vi "Set JSON Value.vi"(8 "error in (no error)":errorcluster, 9 "File Contents":string="{\n    \"SMUResourceName\": \"SMU1\",\n    \"SMUChannels\": \"0\",\n\t\"SMUSourceMode_Sequence\": 1021,\n\t\"SMUOutputFunction_DCCurrent\": 1007,\n    \"SMUSourceTransientResponse_Fast\": 1039,\n    \"SMUCurrent\": 1.0,\n    \"SMUCurrentLevelRange\": 1.0,\n    \"SMUMeasurementSense_Local\": 1008,\n    \"SMUMeasurementApertureTime\": 0.010,\n    \"SMUSourceAdvancedSourceDelay\": 0.000100,\n    \"SMUVoltage\": 6,\n    \"SMUSourceAdvancedSequenceLoopCount\": 571,\n    \"SMUMeasurementAdvancedDCNoiseRejection_Normal\": 1044,\n\t\"SMUSequenceName\": \"MySequence\",\n\t\"SMUStep1_Source_DCCurrent_CurrentLevel\": 1150009,\n\t\"SMUStep2_Measurement_ApertureTime\": 1150058,\n\t\"SMUStep3_Source_Advanced_SourceDelay\": 1150051,\n\t\"SMUSequenceNumberOfSteps\": 3,\n\t\"SMUTriggerFromSwitch_StartDigitalEdge\": \"/SMU/PXI_Trig1\",\n\t\"SMUTriggerFromSwitch_SequenceAdvanceDigitalEdge\": \"/SMU/PXI_Trig1\",\n\t\"SMUTriggerToDMM_SourceCompleteEvent\": 1030,\n\t\"SMUTriggerToDMM_SourceCompleteEvent_Value\": \"/SMU/PXI_Trig2\",\n\t\"SMUTriggerToSwitch_SequenceIterationCompleteEvent\": 1032,\n\t\"SMUTriggerToDMM_SequenceIterationCompleteEvent_Value\": \"/SMU/PXI_Trig0\",\n\t\n\t\"Switch1ResourceName\": \"2526_1\",\n\t\"Switch1Topology\": \"2526/2-Wire 79x1 Mux\",\n\t\"Switch1ScanList\": \"ch70:75->com\",\n\t\n\t\"Switch2ResourceName\": \"SwitchBlock1Dev1\",\n\t\"Switch2Topology\": \"Configured Topology\",\n\t\"Switch2ScanList\": \"[c2->card1r2->c26], [c3->card1r3->c27]; [c6->card1r2->c26], [c7->card1r3->c27]; [c10->card1r2->c26], [c11->card1r3->c27]; [c14->card1r2->c26], [c15->card1r3->c27]; [c18->card1r2->c26], [c19->card1r3->c27]; [c22->card1r2->c26], [c23->card1r3->c27];\",\n\t\n\t\"DMMResourceName\": \"DMM\",\n\t\"DMMFunction_DCVolts\": 0,\n\t\"DMMResolution\": 0.1,\n\t\"DMMRange\": 0.1,\n\t\"DMMTriggerSource_TTL2\": 4,\n\t\"DMMTriggerSlope_RisingEdge\": 0,\n\t\"DMMSampleTrigger_TTL2\": 4,\n\t\"DMMSampleCount\": 0,\n\t\"DMMSampleTriggerSlope_RisingEdge\": 0,\n\t\"DMMApertureTimeUnits_Seconds\": 0,\n\t\"DMMApertureTime\": 0.010,\n\t\"DMMNumberOfAverages\": 1,\n\t\"DMMAutoZero_Off\": 0,\n\t\"DMMADCCalibration_Off\": 0,\n\t\"DMMSettleTime\": 0.0001,\n\t\"DMMControlAction_Commit\": 0,\n\t\n\t\"ApplicationNumberOfWeldChannels\": 6\n}", 10 "Parameter and Value":string="SETCONF=SMUResourceName[[CONFPARAM]]=SMU", 11 "JSON Configuration File (.json)":path=path "C:/Users/chericks/Desktop/JSONtest/labview-grpc-query-server/jsontestfile2.json") -> (0 "error out":errorcluster)   [LabVIEW 2019]
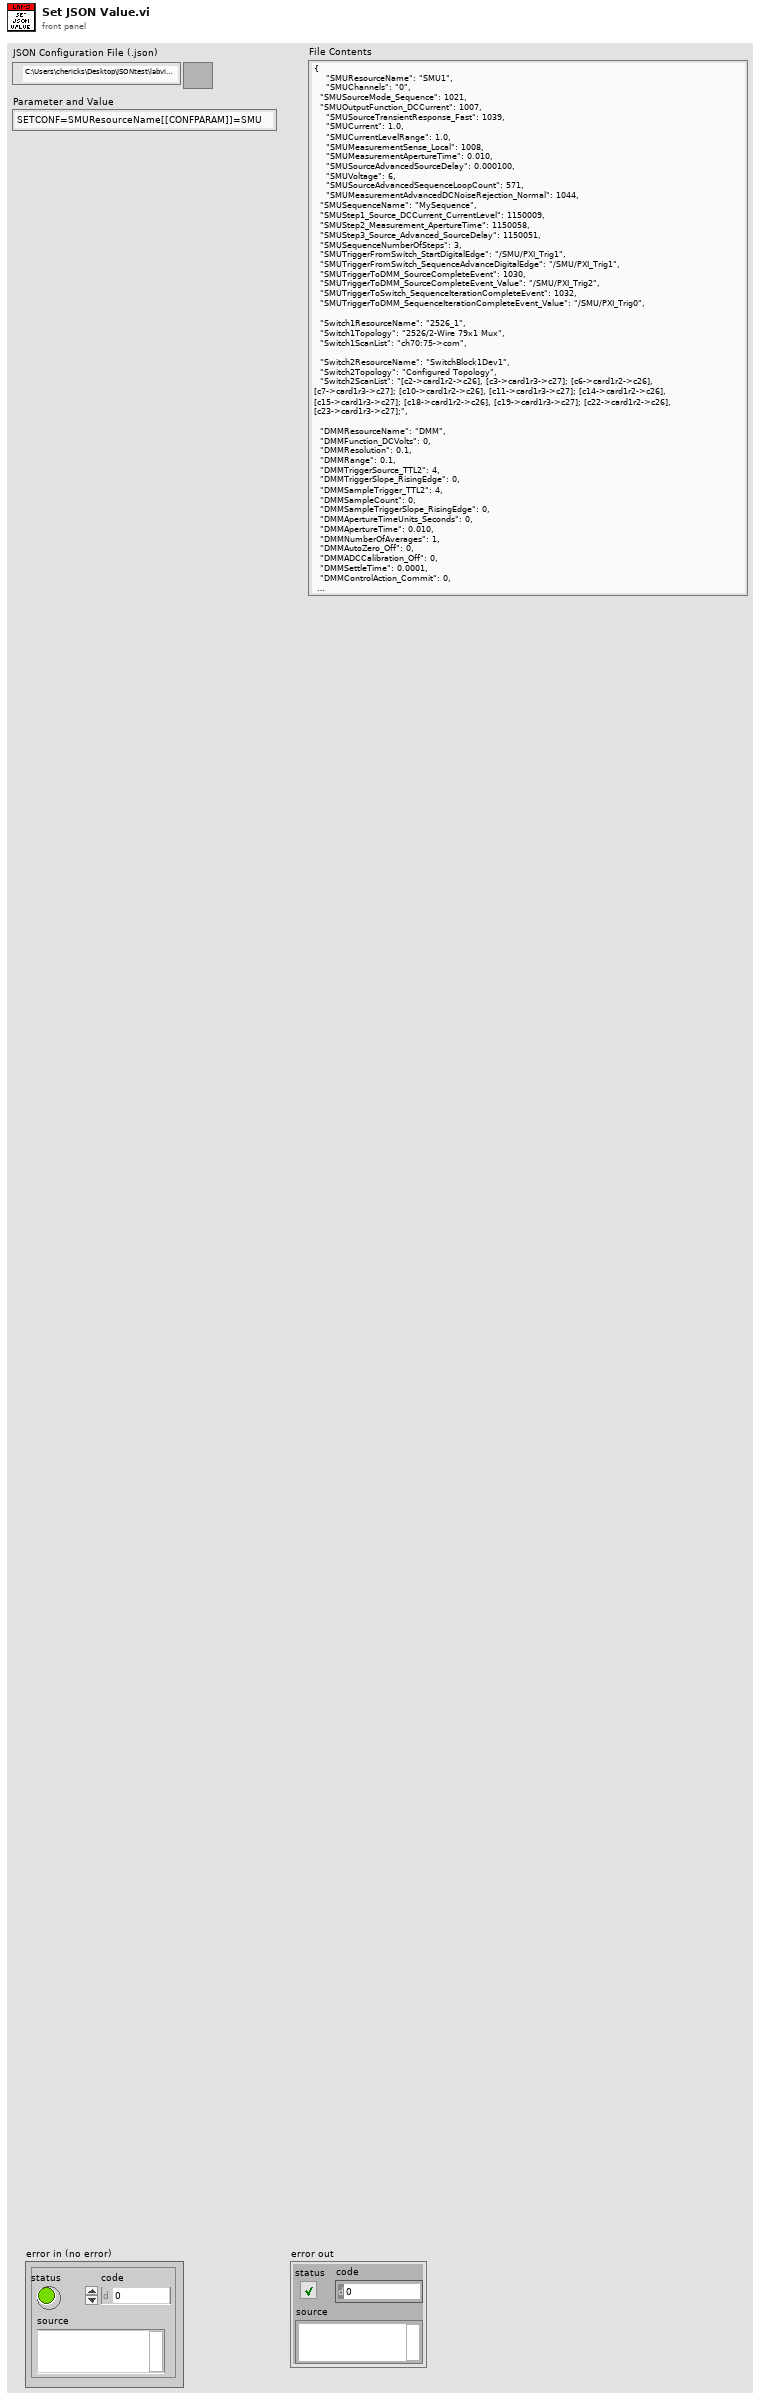
[diagram p1: front panel]
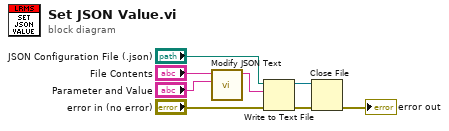
[diagram p0: block diagram]
diagram:
  n1 = call "Modify JSON Text.vi"("Parameter and Value"="Parameter and Value", "JSONtextin"="File Contents") -> ("JSONtextout"=w2:string)  [unwired: 9 in]
  n2 = Write to Text File(file (use dialog)="JSON Configuration File (.json)", text=w2, error in="error in (no error)") -> (refnum out=w5:refnum<file>, error out=w4:errorcluster)  [unwired: 1 in, 1 out]
  n3 = Close File(refnum=w5, error in=w4) -> (error out=→"error out":errorcluster)  [unwired: 1 out]
